vi "Main Page.vi"(8 "error in (no error)":errorcluster, 11 "Node Ptr":T1 format="%.0x") -> (0 "error out":errorcluster)   [LabVIEW 2023, in "Vires VTD System Explorer.lvlib"]
uses:
  Vires VTD System Explorer.lvlib
  <vilib>/NI VeriStand/Custom Device API/Custom Device Item Ref.ctl
  Shared/Input Validation Type.ctl
  <vilib>/NI VeriStand/Custom Device API/Custom Device API.lvlib
  Shared/Vires VTD Shared.lvlib
panel:
  in  "Vires Server IP Address":string
  out "Version":string
  in  "SHDocVw.IWebBrowser2":refnum<k7>(container)
  in  "Header":cluster{"Section Name":string}={"Section Name"="Custom Device Network Settings"}
  in  "Description":string
  in  "Name":string
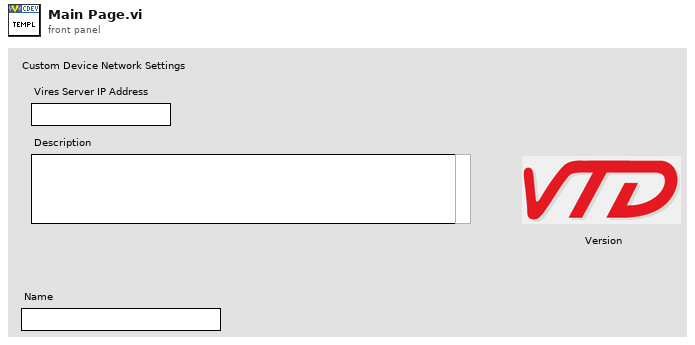
[diagram p1: front panel]
types:
  T1 = typedef "Custom Device API.lvlib/Custom Device Item Ref.ctl" = u64
  T2 = typedef "Vires VTD Shared.lvlib/Network Settings.ctl" = cluster{"IP adress":string, "RDB":cluster{"Protocol":T3, "Tx Port":u16, "Rx Port":u16, "Buffer Size":i32, "Timeout":u16}, "SCP":cluster{"Protocol":T3, "Tx Port":u16, "Rx Port":u16, "Buffer Size":i32, "Timeout":u16}}
  T3 = typedef "Vires VTD Shared.lvlib/Protocol.ctl" = enum16{"UDP", "TCP"}
  T4 = typedef "Custom Device API.lvlib/Custom Device Item Info.ctl" = cluster{"Name":string, "Is Channel":bool, "GUID":string, "Is Waveform":bool}
  T5 = typedef "Vires VTD Shared.lvlib/Input Validation Type.ctl" = enum16{"IP"}
  T6 = typedef "Custom Device API.lvlib/Custom Device Commands.ctl" = enum16{"Default", "Item renamed", "Shutdown", "Dynamic button pressed"}
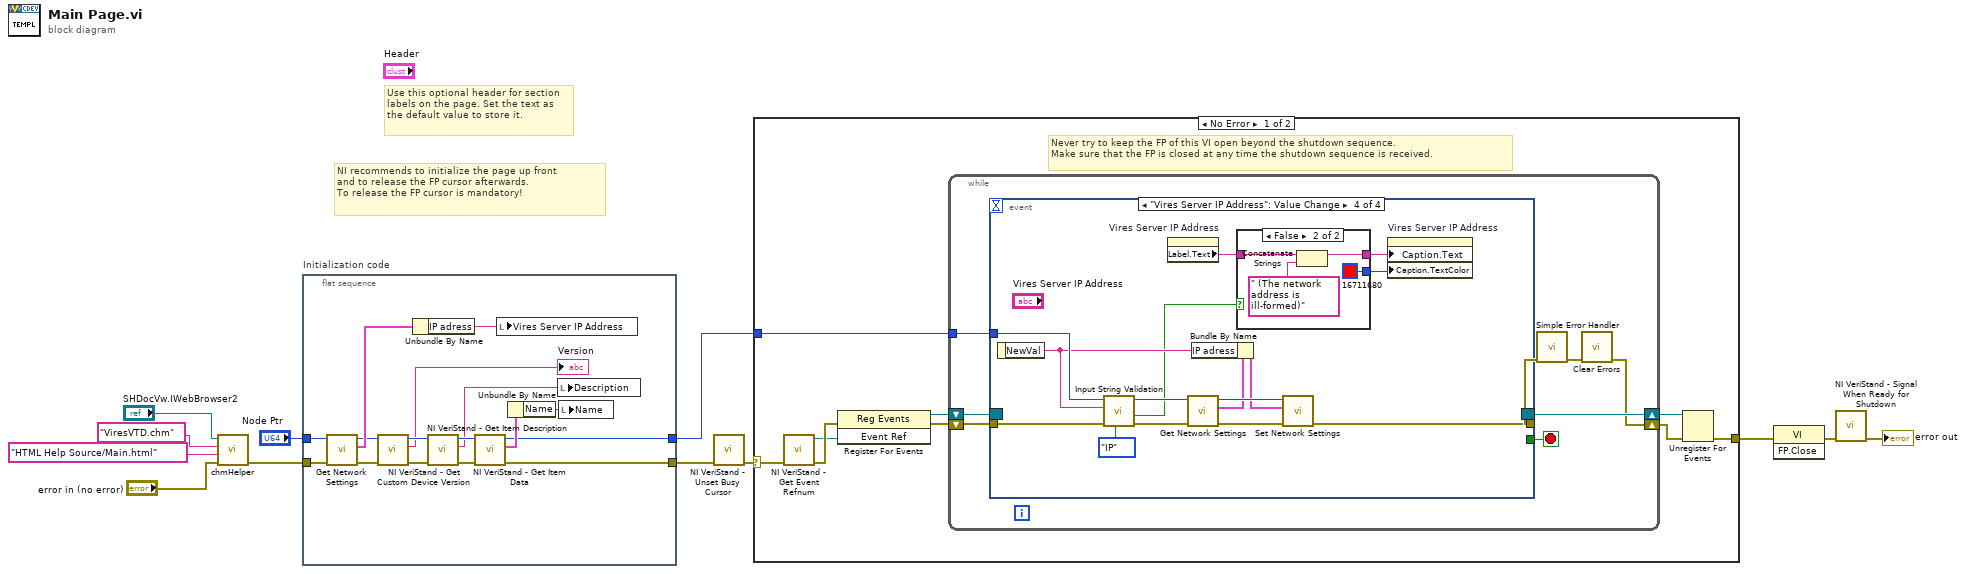
[diagram p0: block diagram]
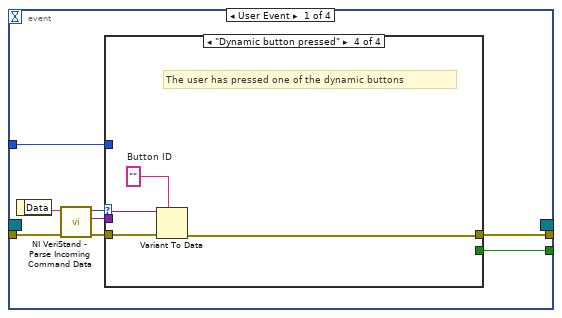
[diagram p2: hidden frame]
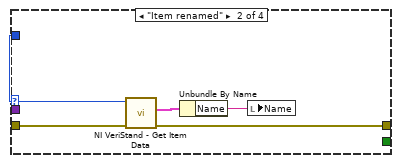
[diagram p4: hidden frame]
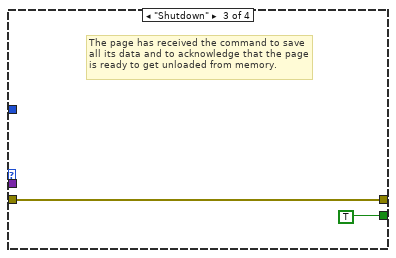
[diagram p5: hidden frame]
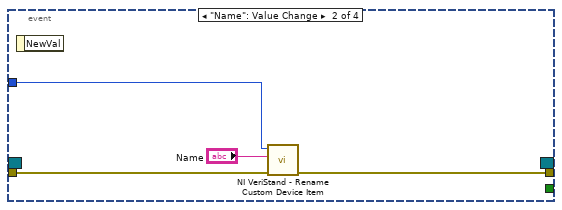
[diagram p6: hidden frame]
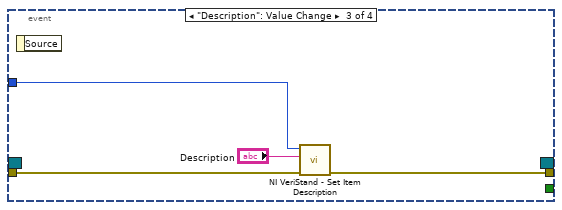
[diagram p7: hidden frame]
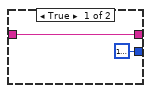
[diagram p8: hidden frame]
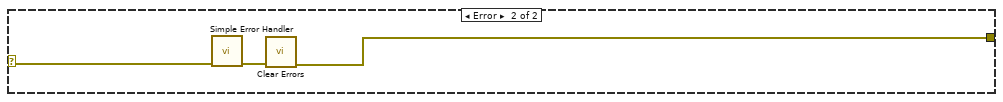
[diagram p9: hidden frame]
diagram:
  # "Use this optional header for section labels on the page. Set the text as the default value to store it."
  # "NI recommends to initialize the page up front\nand to release the FP cursor afterwards.\nTo release the FP cursor is mandatory!"
  n1 = call "chmHelper.vi"("error in (no error)"="error in (no error)", "HTML File"="HTML Help Source/Main.html", "Main CHM File"="ViresVTD.chm" ("HTML File"), "Automation Refnum in"="SHDocVw.IWebBrowser2") -> ("error out"=w4:errorcluster)  [unwired: 7 in]
  n2 = flat-sequence "Initialization code" {
    tunnel: w4 -> [w14]
    tunnel: "Node Ptr" -> [w15]
    tunnel: [w13] -> w8
    tunnel: [w20] -> w6
    frame #0 {
      n3 = call "Get Network Settings.vi"("error in"=w14, "Item Ref in"=w15) -> ("error out"=w16:errorcluster, "Network Settings"=w19:T2, "Item Ref out"=w17:T1)  [unwired: 7 in]
      n4 = call <vilib>:"NI VeriStand - Get Custom Device Version.vi"("error in (no error)"=w16, "Device Ref in"=w17) -> ("error out"=w22:errorcluster, "Value"=→"Version":string, "Device Ref out"=w23:T1)  [unwired: 7 in]
      n5 = Unbundle By Name(w19) -> ("IP adress"=w18:string)
      n6 = call <vilib>:"NI VeriStand - Get Item Description.vi"("error in (no error)"=w22, "Item Ref in"=w23) -> ("error out"=w26:errorcluster, "Description"=w27:string, "Item Ref out"=w28:T1)  [unwired: 7 out]
      n7 = call <vilib>:"NI VeriStand - Get Item Data.vi"("error in (no error)"=w26, "Item Ref in"=w28) -> ("error out"=w13:errorcluster, "Item Info"=w25:T4, "Item Ref out"=w20:T1)  [unwired: 7 out]
      n8 = local write "Vires Server IP Address"(w18) -> ()
      n9 = Unbundle By Name(w25) -> ("Name"=w24:string)
      n10 = local write "Description"(w27) -> ()
      n11 = local write "Name"(w24) -> ()
    }
  }
  n12 = call <vilib>:"NI VeriStand - Unset Busy Cursor.vi"("error in (no error)"=w8) -> ("error out"=w7:errorcluster)  [unwired: 10 out]
  n13 = case shown="No Error" w7 {
    selector: w7 -> [w29 w97]
    tunnel: [w34 w95] -> w12
    tunnel: w6 -> [w30 _]
    frame No Error {
      # "Never try to keep the FP of this VI open beyond the shutdown sequence.\nMake sure that the FP is closed at any time the shutdown sequence is received."
      n14 = call <vilib>:"NI VeriStand - Get Event Refnum.vi"("error in (no error)"=w29) -> ("error out"=w37:errorcluster, "Event Ref"=w33:refnum<user-event>)  [unwired: 9 out]
      n15 = register-events(error in=w37, w33) -> (reference out=w31:refnum<event-registration>, error out=w32:errorcluster)  [unwired: 1 in]
      n16 = while {
        tunnel: w30 -> [w41]
        shift-right: [w38] -> w35
        shift-left: w32 -> [w44]
        shift-right: [w45] -> w36
        shift-left: w31 -> [w43]
        stop <- w42 stop-if-true
        n17 = event shown="[3] \"Vires Server IP Address\": Value Change" {
          selector: w43 -> [_ _ _ _]
          dyn-events: [_ _ _ _] -> w45
          timeout: _ -> [_ _ _ _]
          tunnel: w44 -> [w53 w69 w72 w80]
          tunnel: [w49 _ _ _] -> w42
          tunnel: [w48 w68 w71 w79] -> w40
          tunnel: w41 -> [w47 w67 w73 w81]
          event User Event {
            n18 = event-data() -> ("Data"=w52:string)  [unwired: 1 out]
            n19 = call <vilib>:"NI VeriStand - Parse Incoming Command Data.vi"("error in (no error)"=w53, "Incoming data"=w52) -> ("error out"=w51:errorcluster, "Outgoing data"=w46:variant, "Action"=w50:T6)  [unwired: 7 out]
            n20 = case shown="\"Dynamic button pressed\"" w50 {
              tunnel: w51 -> [w54 w59 w60 w65]
              tunnel: [_ _ TRUE _] -> w49
              tunnel: [w54 w57 w60 w62] -> w48
              tunnel: w47 -> [_ w55 _ _]
              tunnel: w46 -> [_ _ _ w64]
              frame "Default", Default {
              }
              frame "Item renamed" {
                n21 = call <vilib>:"NI VeriStand - Get Item Data.vi"("error in (no error)"=w59, "Item Ref in"=w55) -> ("error out"=w57:errorcluster, "Item Info"=w58:T4)  [unwired: 8 out]
                n22 = Unbundle By Name(w58) -> ("Name"=w56:string)
                n23 = local write "Name"(w56) -> ()
              }
              frame "Shutdown" {
                # "The page has received the command to save all its data and to acknowledge that the page is ready to get unloaded from memory."
              }
              frame "Dynamic button pressed" {
                w63 = ""  # Button ID
                # "The user has pressed one of the dynamic buttons"
                n24 = Variant To Data(error in=w65, type=w63, Variant=w64) -> (error out=w62:errorcluster)  [unwired: 1 out]
              }
            }
          }
          event "Name": Value Change {
            n25 = event-data() -> ()  [unwired: 2 out]
            n26 = call <vilib>:"NI VeriStand - Rename Custom Device Item.vi"("error in (no error)"=w69, "New Name"="Name", "Item Ref in"=w67) -> ("error out"=w68:errorcluster)  [unwired: 1 in, 7 out]
          }
          event "Description": Value Change {
            n27 = event-data() -> ()  [unwired: 2 out]
            n28 = call <vilib>:"NI VeriStand - Set Item Description.vi"("error in (no error)"=w72, "Description"="Description", "Item Ref in"=w73) -> ("error out"=w71:errorcluster)  [unwired: 8 out]
          }
          event "Vires Server IP Address": Value Change {
            n29 = event-data() -> ("NewVal"=w78:string)  [unwired: 1 out]
            n30 = call "Input String Validation.vi"("Input Type"=Input_Validation_Type."IP", "Error In"=w80, "String to check"=w78, "Item Ref in"=w81) -> ("Error Out"=w83:errorcluster, "Valid?"=w74:bool, "Item Ref out"=w82:T1)  [unwired: 4 in, 1 out]
            n31 = property on="Vires Server IP Address" class="Str"() -> ("Label.Text"=w76:string)  [unwired: 2 in, 2 out]
            n32 = call "Get Network Settings.vi"("error in"=w83, "Item Ref in"=w82) -> ("error out"=w85:errorcluster, "Network Settings"=w87:T2, "Item Ref out"=w88:T1)  [unwired: 7 in]
            n33 = Bundle By Name(cluster=w87, "IP adress"=w78) -> (w86:T2)
            n34 = case shown="False" w74 {
              tunnel: [u32 16777222 u32 16711680] -> w75
              tunnel: [w89 w92] -> w77
              tunnel: w76 -> [w89 w93]
              frame True {
              }
              frame False {
                n35 = Concatenate Strings(w93, " (The network address is ill-formed)" ("string")) -> (w92:string)
              }
            }
            n36 = call "Set Network Settings.vi"("error in"=w85, "Network Settings"=w86, "Item Ref in"=w88) -> ("error out"=w79:errorcluster)  [unwired: 7 in, 1 out]
            n37 = property on="Vires Server IP Address" class="Str"("Caption.Text"=w77, "Caption.TextColor"=w75) -> ()  [unwired: 2 in, 2 out]
          }
        }
        n38 = call <vilib>:"Simple Error Handler.vi"("error in (no error)"=w40) -> ("error out"=w39:errorcluster)  [unwired: 1 in, 7 out]
        n39 = call <vilib>:"Clear Errors.vi"("error in (no error)"=w39) -> ("error out"=w38:errorcluster)  [unwired: 1 in, 5 out]
      }
      n40 = Unregister For Events(event registration refnum=w36, error in=w35) -> (error out=w34:errorcluster)
    }
    frame Error {
      n41 = call <vilib>:"Simple Error Handler.vi"("error in (no error)"=w97) -> ("error out"=w96:errorcluster)  [unwired: 1 in, 7 out]
      n42 = call <vilib>:"Clear Errors.vi"("error in (no error)"=w96) -> ("error out"=w95:errorcluster)  [unwired: 1 in, 5 out]
    }
  }
  n43 = invoke class="VI" method="FP.Close"(error in=w12) -> (error out=w11:errorcluster)  [unwired: 2 in, 2 out]
  n44 = call <vilib>:"NI VeriStand - Signal When Ready for Shutdown.vi"("error in (no error)"=w11) -> ("error out"=→"error out":errorcluster)  [unwired: 10 out]
